vi "Test_Device_Info_Panel.vi"() -> ()   [LabVIEW 2024]
uses:
  RPC Messages/rfcontrol_DeviceInformationRequest.ctl
  FlexSDR_gRPC_client.lvlib
panel:
  out "error out":errorcluster
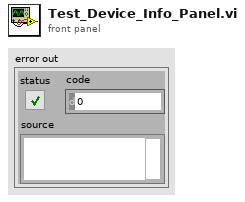
[diagram p1: front panel]
types:
  T1 = typedef "FlexSDR_gRPC_client.lvlib/rfcontrol_DeviceInformationRequest.ctl" = cluster{"device_id":string, "error_queue_populate":bool}
  T2 = typedef "grpc-lvsupport-release.lvlib/grpcId.ctl" = u64
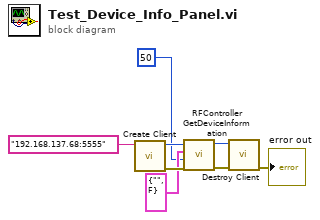
[diagram p0: block diagram]
diagram:
  n1 = call "Create Client.vi"("address"="192.168.137.68:5555") -> ("error out"=w7:errorcluster, "gRPC ID Out"=w5:T2)  [unwired: 9 in]
  n2 = call "RFController GetDeviceInformation.vi"("error in"=w7, "timeout (ms)"=50, "Request Data"=T1 {"device_id"="", "error_queue_populate"=FALSE}, "gRPC ID"=w5) -> ("error out"=w4:errorcluster, "gRPC ID out"=w3:T2)  [unwired: 5 in, 1 out]
  n3 = call "Destroy Client.vi"("error in"=w4, "gRPC ID"=w3) -> ("error out"=→"error out":errorcluster)  [unwired: 9 in]
